vi "Get Data from LUT.vi"(8 "error in":errorcluster, 10 "Keys":string[](array[string]), 11 "Variant In":variant) -> (0 "error out":errorcluster, 2 "Values":string[](array[string]), 3 "Variant Out":variant)   [LabVIEW 2019, in "Inset.lvclass"]
uses:
  Inset.lvclass
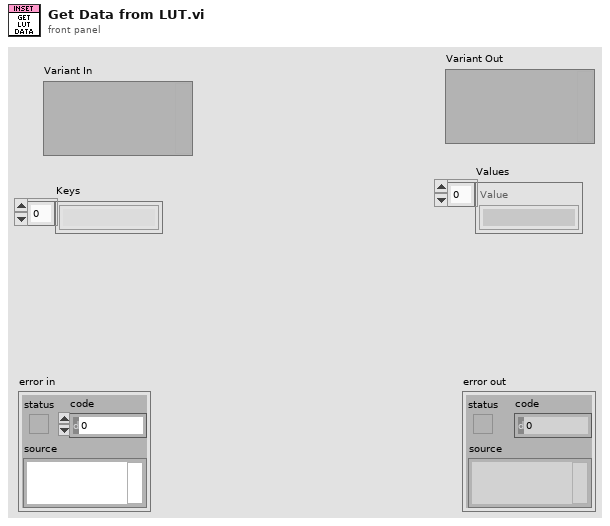
[diagram p1: front panel]
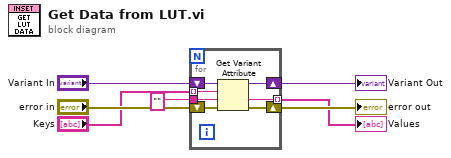
[diagram p0: block diagram]
diagram:
  n1 = for {
    shift-right: [w13] -> w6
    shift-left: "Variant In" -> [w14]
    shift-right: [w11] -> w4
    shift-left: "error in" -> [w12]
    tunnel: "Keys" -> [w10] mode=indexing
    tunnel: "" -> [w9]
    tunnel: [w8] -> w1 mode=indexing
    n2 = Get Variant Attribute(Variant=w14, name=w10, default value (empty Variant)=w9, error in=w12) -> (duplicate Variant=w13:variant, value=w8:string, error out=w11:errorcluster)  [unwired: 1 out]
  }
  "error out" <- w4
  "Variant Out" <- w6
  "Values" <- w1
